vi "getRect.vi"(9 "Y":dbl, 10 "X":dbl, 11 "Offset":dbl) -> (0 "B":dbl, 1 "R":dbl, 2 "T":dbl, 3 "L":dbl)   [LabVIEW 2013]
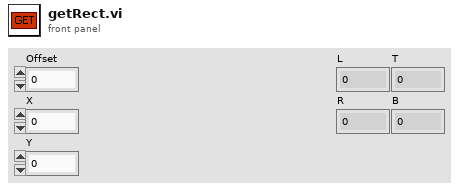
[diagram p1: front panel]
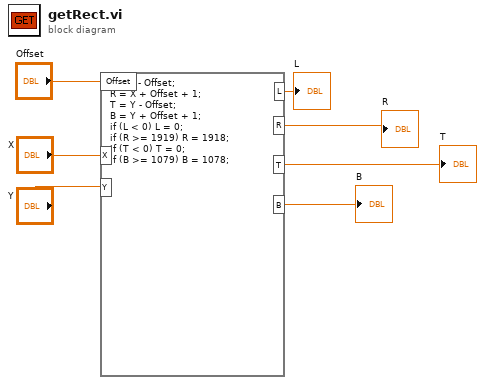
[diagram p0: block diagram]
diagram:
  n1 = formula code="L = X - Offset;\nR = X + Offset + 1;\nT = Y - Offset;\nB = Y + Offset + 1;\nif (L < 0) L = 0;\nif (R >= 1919) R = 1918;\nif (T < 0) T = 0;\nif (B >= 1079) B = 1078;"("X"="X", "Y"="Y", "Offset"="Offset") -> ("L"=→"L":dbl, "R"=→"R":dbl, "T"=→"T":dbl, "B"=→"B":dbl)
